vi "ATM_FP.Calculate_CheckSum.vi"(11 "DataPacket":string="ï\u0001ÿÿÿÿ\u0001\u0000\u0003\u0001\u0000\u0005") -> (1 "Checksum":string, 3 "DataPacket+Checksum":string)   [LabVIEW 2020]
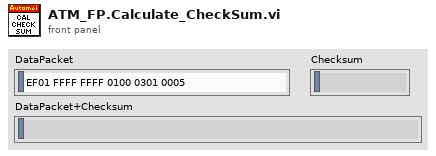
[diagram p1: front panel]
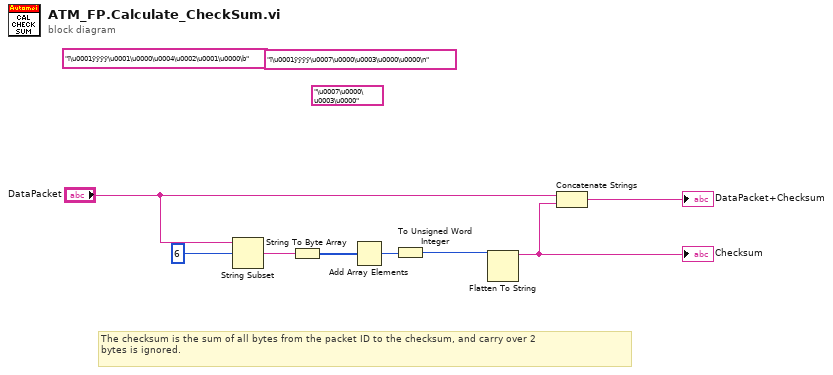
[diagram p0: block diagram]
diagram:
  (unwired) "ï\u0001ÿÿÿÿ\u0007\u0000\u0003\u0000\u0000\n" ("read buffer 2")
  (unwired) "ï\u0001ÿÿÿÿ\u0001\u0000\u0004\u0002\u0001\u0000\b" ("读取缓冲区输入")
  (unwired) "\u0007\u0000\u0003\u0000" ("y")
  # "The checksum is the sum of all bytes from the packet ID to the checksum, and carry over 2\nbytes is ignored."
  n1 = String Subset(string="DataPacket", offset (0)=6) -> (substring=w7:string)  [unwired: 1 in]
  n2 = String To Byte Array(string=w7) -> (unsigned byte array=w6:u8[])
  n3 = Add Array Elements(numeric array=w6) -> (sum=w5:u8)
  n4 = To Unsigned Word Integer(number=w5) -> (unsigned 16bit integer=w4:u16)
  n5 = Flatten To String(anything=w4) -> (data string=w2:string)  [unwired: 3 in, 2 out]
  "Checksum" <- w2
  n6 = Concatenate Strings("DataPacket", w2) -> (→"DataPacket+Checksum":string)
